vi "FindAB.vi"(9 "# linear fit points":i32, 10 "# pts of A":i32, 11 "Normalized angles":cluster{i32, "Sample time":dbl, dbl[]}[](graph)) -> (0 "B":dbl, 1 "A":dbl, 2 "A values":dbl[](array[numeric]), 3 "Closeup":dbl[][](array[numeric]), 5 "B values":dbl[](array[numeric]))   [LabVIEW 2022 SP3]
uses:
  <vilib>/Analysis/baseanly.llb/Mean (DBL).vi
  <vilib>/Analysis/NI_AALPro.lvlib
  <vilib>/Analysis/NI_AALBase.lvlib
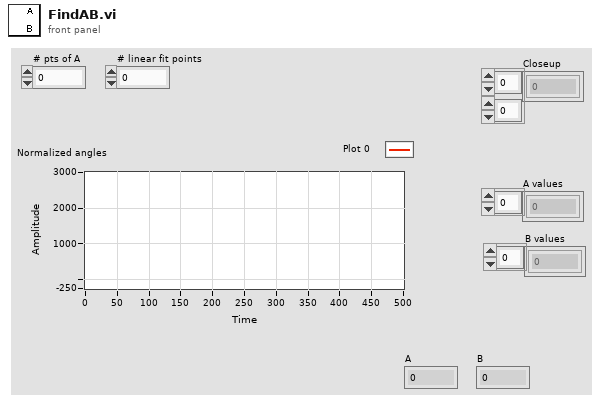
[diagram p1: front panel]
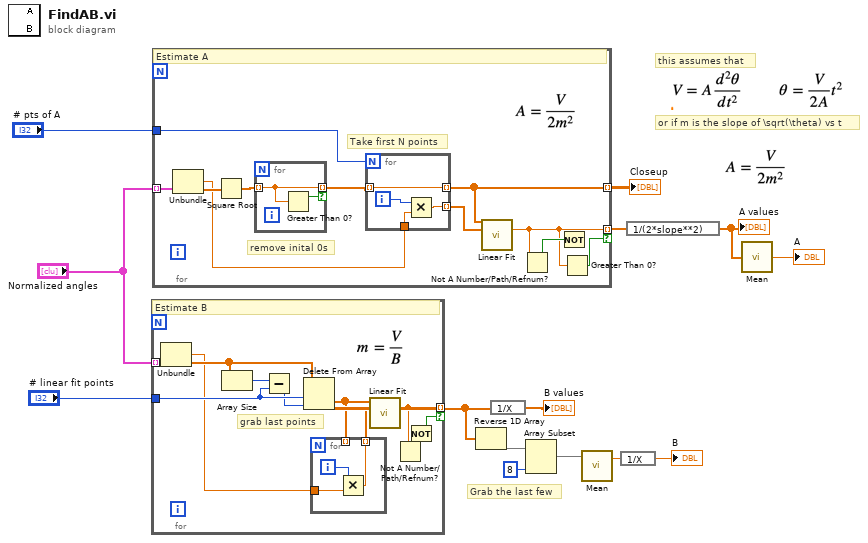
[diagram p0: block diagram]
diagram:
  # "or if m is the slope of \\sqrt(\\theta) vs t"
  # "this assumes that"
  # "Grab the last few"
  n1 = for {
    tunnel: "Normalized angles" -> [w23] mode=indexing
    tunnel: [w17] -> w12 mode=indexing if=w15
    tunnel: "# linear fit points" -> [w21]
    # "grab last points"
    # "Estimate B"
    n2 = Unbundle(w23) -> ("Sample time"=w18:dbl, w19:dbl[])  [unwired: 1 out]
    n3 = Array Size(array=w19) -> (size(s)=w22:i32)
    n4 = Subtract(x=w22, y=w21) -> (x-y=w20:i32)
    n5 = Delete From Array(array=w19, length=w21, index=w20) -> (deleted portion=w25:dbl[])  [unwired: 1 out]
    n6 = for {
      tunnel: w25 -> [_] mode=indexing
      tunnel: [w26] -> w24 mode=indexing
      tunnel: w18 -> [w27]
      i -> [w28]
      n7 = Multiply(x=w28, y=w27) -> (x*y=w26:dbl)
    }
    n8 = call <vilib>:"Linear Fit.vi"("Y"=w25, "X"=w24) -> ("slope"=w17:dbl)  [unwired: 9 in, 4 out]
    n9 = Not A Number/Path/Refnum?(number/path/refnum=w17) -> (NaN/Path/Refnum?=w16:bool)
    n10 = Not(x=w16) -> (.not. x?=w15:bool)
  }
  n11 = for {
    tunnel: "Normalized angles" -> [w34] mode=indexing
    tunnel: [w37] -> w1 mode=indexing
    tunnel: [w31] -> w8 mode=indexing if=w30
    tunnel: "# pts of A" -> [w29]
    # "remove inital 0s"
    # "Take first N points"
    # "Estimate A"
    n12 = Unbundle(w34) -> ("Sample time"=w32:dbl, w33:dbl[])  [unwired: 1 out]
    n13 = Square Root(x=w33) -> (sqrt(x)=w38:dbl[])
    n14 = for {
      tunnel: w38 -> [w45] mode=indexing
      tunnel: [w45] -> w35 mode=indexing if=w44
      n15 = Greater Than 0?(x=w45) -> (x > 0?=w44:bool)
    }
    n16 = for {
      N: w29 -> [_]
      tunnel: [w40] -> w39 mode=indexing
      tunnel: w35 -> [w43] mode=indexing
      tunnel: [w43] -> w37 mode=indexing
      tunnel: w32 -> [w41]
      i -> [w42]
      n17 = Multiply(x=w42, y=w41) -> (x*y=w40:dbl)
    }
    n18 = call <vilib>:"Linear Fit.vi"("Y"=w37, "X"=w39) -> ("slope"=w31:dbl)  [unwired: 9 in, 4 out]
    n19 = Not A Number/Path/Refnum?(number/path/refnum=w31) -> (NaN/Path/Refnum?=w36:bool)
    n20 = Not(x=w36) -> ()  [unwired: 1 out]
    n21 = Greater Than 0?(x=w31) -> (x > 0?=w30:bool)
  }
  "Closeup" <- w1
  n22 = Reverse 1D Array(array=w12) -> (reversed array=w2:dbl[])
  n23 = expression code="1/X"(w12) -> (→"B values":dbl[])
  n24 = Array Subset(array=w2, length=8) -> (w5:dbl[])  [unwired: 1 in]
  n25 = call-poly <vilib>:"Mean.vi"("X"=w5) -> ("mean"=w4:dbl)  [unwired: 1 out]
  n26 = expression code="1/X"(w4) -> (→"B":dbl)
  n27 = expression code="1/(2*slope**2)"(w8) -> (w9:dbl[])
  "A values" <- w9
  n28 = call-poly <vilib>:"Mean.vi"("X"=w9) -> ("mean"=→"A":dbl)  [unwired: 1 out]
